vi "ShiftPicture.vi"(5 "y_Shift":i16, 7 "x_Shift":i16, 10 "y_Index":i16, 11 "x_Index":i16) -> (2 "y_index_shifted":i16, 3 "x_index_shifted":i16)   [LabVIEW 2019, in "VGA.lvlib"]
uses:
  VGA.lvlib
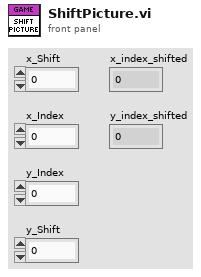
[diagram p1: front panel]
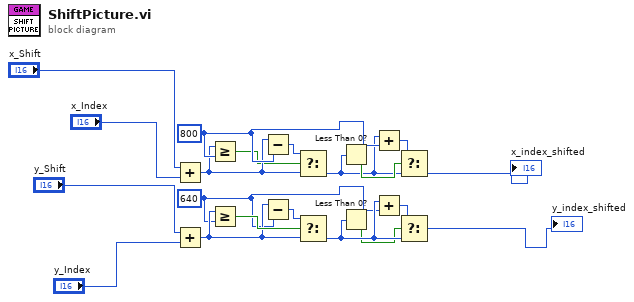
[diagram p0: block diagram]
diagram:
  w13 = i16 640 ("y")
  w7 = i16 800 ("y")
  n1 = Add(x="x_Shift", y="x_Index") -> (x+y=w4:i16)
  n2 = Add(x="y_Shift", y="y_Index") -> (x+y=w16:i16)
  n3 = Greater Or Equal?(x=w4, y=w7) -> (x >= y?=w3:bool)
  n4 = Greater Or Equal?(x=w16, y=w13) -> (x >= y?=w17:bool)
  n5 = Subtract(x=w4, y=w7) -> (x-y=w5:i16)
  n6 = Subtract(x=w16, y=w13) -> (x-y=w15:i16)
  n7 = Select(t=w5, s=w3, f=w4) -> (s? t:f=w6:i16)
  n8 = Select(t=w15, s=w17, f=w16) -> (s? t:f=w14:i16)
  n9 = Less Than 0?(x=w6) -> (x < 0?=w8:bool)
  n10 = Less Than 0?(x=w14) -> (x < 0?=w12:bool)
  n11 = Add(x=w6, y=w7) -> (x+y=w9:i16)
  n12 = Add(x=w14, y=w13) -> (x+y=w11:i16)
  n13 = Select(t=w9, s=w8, f=w6) -> (s? t:f=→"x_index_shifted":i16)
  n14 = Select(t=w11, s=w12, f=w14) -> (s? t:f=→"y_index_shifted":i16)
